vi "CONFIG WINDOWS.vi"() -> ()   [LabVIEW 2009]
uses:
  Valores configuracion test.ctl
panel:
  in  "Config Test":T1=[{"Vin Rate Scan"=[0, 1, 2, 3, 4, 5, 6, 7, 8, 9], "Vasic"=3.3, "Vin Rate Adders"=[0, 1], "Test Max PN Min NP?"=TRUE, "Pattern Max PN Min NP"={"Max P inferior"=1.888, "Max P superior"=2.177000045776367, "Min N superior"=0.818, "Min N inferior"=0.73, "Max N superior"=1.475, "Max N inferior"=1.322, "Min P inferior "=1.321, "Min P superior"=1.474}, "Test Rate Scan?"=TRUE, "Test Rate Scan Adders? 2"=TRUE, "Test offset analog?"=TRUE, "Test offset digital?"=TRUE}, {"Vin Rate Scan"=[0, 3], "Vasic"=3.2, "Vin Rate Adders"=[0, 1], "Test Max PN Min NP?"=TRUE, "Pattern Max PN Min NP"={"Max P inferior"=1.888, "Max P superior"=2.177000045776367, "Min N superior"=0.818, "Min N inferior"=0.73, "Max N superior"=1.475, "Max N inferior"=1.322, "Min P inferior "=1.321, "Min P superior"=1.474}, "Test Rate Scan?"=TRUE, "Test Rate Scan Adders? 2"=TRUE, "Test offset analog?"=TRUE, "Test offset digital?"=TRUE}, {"Vin Rate Scan"=[0, 3], "Vasic"=3.1, "Vin Rate Adders"=[0, 1], "Test Max PN Min NP?"=TRUE, "Pattern Max PN Min NP"={"Max P inferior"=1.888, "Max P superior"=2.177000045776367, "Min N superior"=0.818, "Min N inferior"=0.73, "Max N superior"=1.475, "Max N inferior"=1.322, "Min P inferior "=1.321, "Min P superior"=1.474}, "Test Rate Scan?"=TRUE, "Test Rate Scan Adders? 2"=TRUE, "Test offset analog?"=TRUE, "Test offset digital?"=TRUE}, {"Vin Rate Scan"=[0, 3], "Vasic"=3.0, "Vin Rate Adders"=[0, 1], "Test Max PN Min NP?"=TRUE, "Pattern Max PN Min NP"={"Max P inferior"=1.888, "Max P superior"=2.177000045776367, "Min N superior"=0.818, "Min N inferior"=0.73, "Max N superior"=1.475, "Max N inferior"=1.322, "Min P inferior "=1.321, "Min P superior"=1.474}, "Test Rate Scan?"=TRUE, "Test Rate Scan Adders? 2"=TRUE, "Test offset analog?"=TRUE, "Test offset digital?"=TRUE}] {"Pattern Max PN Min NP"."Min P superior" format="%.3g"; "Pattern Max PN Min NP"."Min P inferior" format="%.3g"; "Pattern Max PN Min NP"."Max N inferior" format="%.3g"; "Pattern Max PN Min NP"."Max N superior" format="%.3g"; "Pattern Max PN Min NP"."Min N inferior" format="%.3g"; "Pattern Max PN Min NP"."Min N superior" format="%.3g"; "Pattern Max PN Min NP"."Max P superior" format="%.3g"; "Pattern Max PN Min NP"."Max P inferior" format="%.3g"; "Vasic" min=2.8 max=3.8 step=0.01 format="%.2g"}
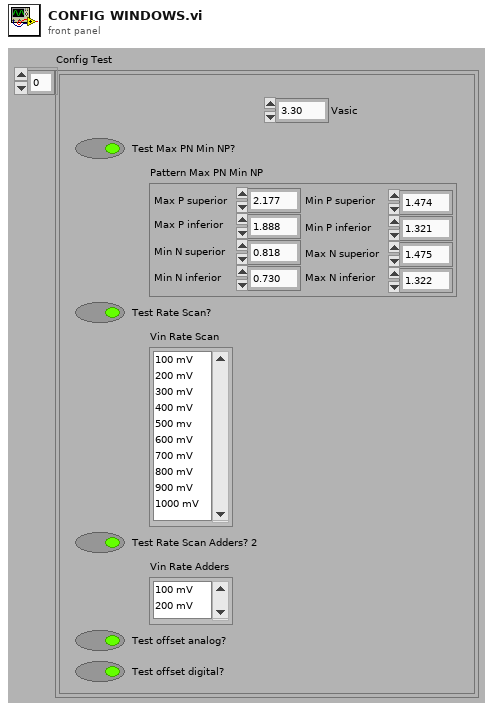
[diagram p1: front panel]
types:
  T1 = typedef "Valores configuracion test.ctl" = cluster{"Vin Rate Scan":i32[], "Vasic":dbl, "Vin Rate Adders":i32[], "Test Max PN Min NP?":bool, "Pattern Max PN Min NP":cluster{"Max P inferior":dbl, "Max P superior":dbl, "Min N superior":dbl, "Min N inferior":dbl, "Max N superior":dbl, "Max N inferior":dbl, "Min P inferior ":dbl, "Min P superior":dbl}, "Test Rate Scan?":bool, "Test Rate Scan Adders? 2":bool, "Test offset analog?":bool, "Test offset digital?":bool}[]
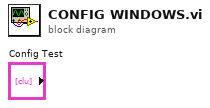
[diagram p0: block diagram]
diagram:
